vi "Rotate Picture Control.vi"() -> ()   [LabVIEW 2023]
doc: "Uses the Picture to 2D Pixmap VI with the Rotate Pixmap VI to rotate the image of a picture control."
uses:
  Rotate.llb/rotate 24bit.vi
panel:
  in  "Fill Color":u32(colorbox)
  in  "Size":cluster{"Width":u32, "Height":u32}={"Width"=212, "Height"=172}
  in  "Original Picture":picture
  in  "Maintain Center Position?":bool
  in  "Rotation Angle (degrees)":dbl=30.0 format="%.2f"
  out "Rotated Picture":picture
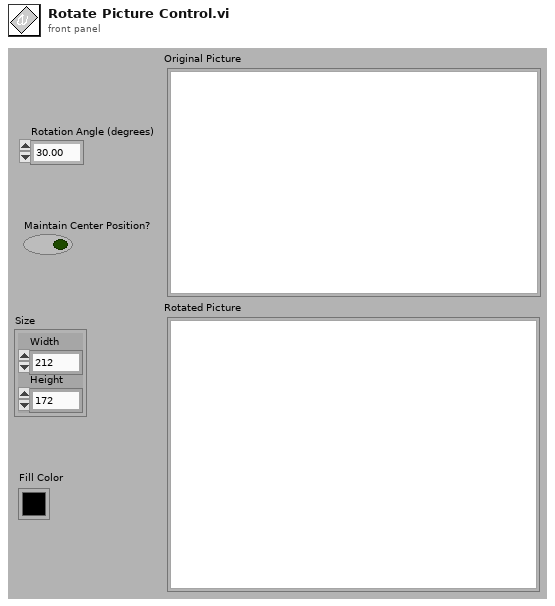
[diagram p1: front panel]
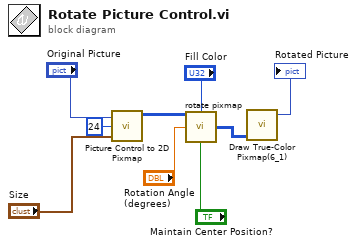
[diagram p0: block diagram]
diagram:
  n1 = call "Picture Control to 2D Pixmap.vi"("Picture"="Original Picture", "image depth"=u8 24, "Draw Area Size"="Size") -> ("24-bit"=w9:u32[][])  [unwired: 1 in, 3 out]
  n2 = call-poly "rotate pixmap.vi"("Color Table Index of Fill Color"="Fill Color", "Maintain Center Position?"="Maintain Center Position?", "Rotation Angle (degrees)"="Rotation Angle (degrees)", "Pixmap"=w9) -> ("Rotated Pixmap"=w6:u32[][])
  n3 = call <vilib>:"Draw True-Color Pixmap(6_1).vi"("data (RGB format)"=w6) -> ("new picture"=→"Rotated Picture":picture)  [unwired: 8 in]
